vi "VCS Get Device Name Selection.vi"(0 "device in":T1, 5 "StartOfSelection":i32, 11 "error in (no error)":errorcluster) -> (4 "device out":T1={"deviceName"="EPOS2", "protocolStackName"="", "interfaceName"="", "portName"=""}, 6 "endOfSelection":i32, 8 "deviceNameSel":string, 15 "error out":errorcluster)   [LabVIEW 2019, in "maxonEPOS.lvlib"]
doc: "<B>VCS GetDeviceNameSelection</B> returns all available device names."
uses:
  Examples/maxonEPOS.lvlib
  Resources/EposCmd.dll
  Resources/EposCmd64.dll
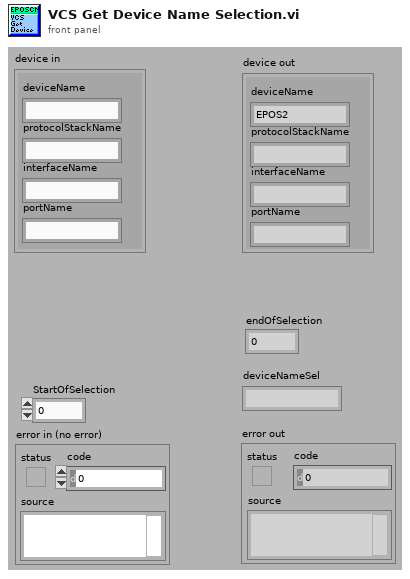
[diagram p1: front panel]
types:
  T1 = cluster{"deviceName":string, "protocolStackName":string, "interfaceName":string, "portName":string}
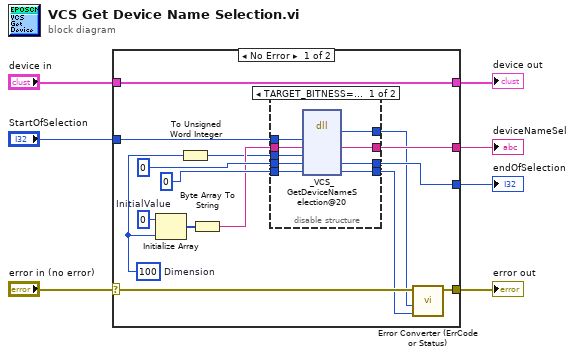
[diagram p0: block diagram]
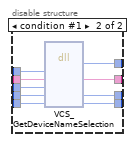
[diagram p2: hidden frame]
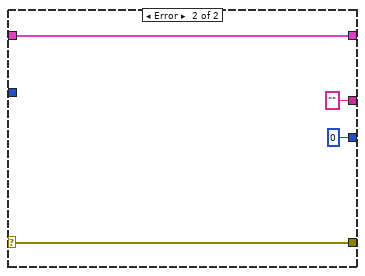
[diagram p3: hidden frame]
diagram:
  n1 = case shown="No Error" "error in (no error)" {
    selector: "error in (no error)" -> [w19 w44]
    tunnel: [w18 w44] -> w6
    tunnel: "StartOfSelection" -> [w22 _]
    tunnel: [w21 "" ("pDeviceNameSel")] -> w4
    tunnel: [w20 0 ("pEndOfSelection")] -> w3
    tunnel: "device in" -> [w16 w43]
    tunnel: [w16 w43] -> w1
    frame No Error {
      w12 = u8 0  # InitialValue
      w8 = 100  # Dimension
      n2 = Initialize Array(w12, w8) -> (w13:u8[])
      n3 = To Unsigned Word Integer(number=w8) -> (unsigned 16bit integer=w9:u16)
      n4 = Byte Array To String(unsigned byte array=w13) -> (string=w10:string)
      n5 = disable-structure shown="TARGET_BITNESS==32, Standard" {
        disable-tunnel: w22 -> [w31 w40]
        disable-tunnel: [w30 w39] -> w21
        disable-tunnel: [w29 w38] -> w20
        disable-tunnel: [w28 w37] -> w17
        disable-tunnel: u32 0 ("pErrorCode") -> [w27 w36]
        disable-tunnel: 0 ("pEndOfSelection") -> [w26 w35]
        disable-tunnel: [w25 w34] -> w11
        disable-tunnel: w10 -> [w24 w33]
        disable-tunnel: w9 -> [w23 w32]
        frame condition #0 (active) {
          n6 = dll-call lib="C:/workspace/project/scancon/sw/SSI_Tool/InstrumentsInterfaces/Motordriver/maxon EPOS/Resources/EposCmd.*" fn="_VCS_GetDeviceNameSelection@20"("StartOfSelection"=w31, "pDeviceNameSel"=w24, "MaxStrSize"=w23, "pEndOfSelection"=w26, "pErrorCode"=w27) -> (w25:i32, "pDeviceNameSel"=w30:string, "pEndOfSelection"=w29:i32, "pErrorCode"=w28:u32)  [unwired: 5 in, 2 out]
        }
        frame condition #1 {
          n7 = dll-call lib="C:/setup/Resources/EposCmd64.dll" fn="VCS_GetDeviceNameSelection" ("EposCmd.dll:_VCS_GetDeviceNameSelection@20")("StartOfSelection"=w40, "pDeviceNameSel"=w33, "MaxStrSize"=w32, "pEndOfSelection"=w35, "pErrorCode"=w36) -> ("Rückgabetyp"=w34:i32, "pDeviceNameSel"=w39:string, "pEndOfSelection"=w38:i32, "pErrorCode"=w37:u32)  [unwired: 5 in, 2 out]
        }
      }
      n8 = call "Error Converter (ErrCode or Status).vi"("error code"=w17, "return type"=w11, "error in (no error)"=w19) -> ("error out"=w18:errorcluster)  [unwired: 7 in]
    }
    frame Error {
    }
  }
  "deviceNameSel" <- w4
  "endOfSelection" <- w3
  "error out" <- w6
  "device out" <- w1
